vi "global.vi"() -> ()   [LabVIEW 2017]
panel:
  in  "global":dbl
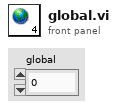
[diagram p1: front panel]
diagram:
